vi "Relay Controller.vi"(0 "TSM Context":T2, 7 "Relays":string[](array[string]), 11 "error in":errorcluster) -> (15 "error out":errorcluster)   [LabVIEW 2019]
doc: "This VI is used for toggling 2567, 6368 and 6571 based relays."
uses:
  <vilib>/NI_TestStand_SemiconductorModule/NI_TestStand_Semiconductor_Module.lvlibp/PinMap/General/SemiconductorModuleContext.ctl
  <vilib>/NI_TestStand_SemiconductorModule/NI_TestStand_Semiconductor_Module.lvlibp/1abvi3w/instr.lib/niSwitch/niswitch.llb/niSwitch Relay Action.ctl
  <vilib>/Utility/error.llb/whitespace.ctl
  <vilib>/DAQmx/write.llb/DAQmx Write (Digital 2D Bool NChan 1Samp NLine).vi
  <vilib>/DAQmx/miscellaneous.llb/DAQmx Fill In Error Info.vi
  <vilib>/NI_TestStand_SemiconductorModule/NI_TestStand_Semiconductor_Module.lvlibp
  <instrlib>/niDigital/niDigital.llb/niDigital Write Static Pin State.ctl
  <vilib>/DAQmx/write.llb/DAQmx Write (Digital Bool 1Line 1Point).vi
panel:
  in  "Relay Control":T1=21 caption="relay action (Close Relay)" items=["Open Relay"=20, "Close Relay"=21]
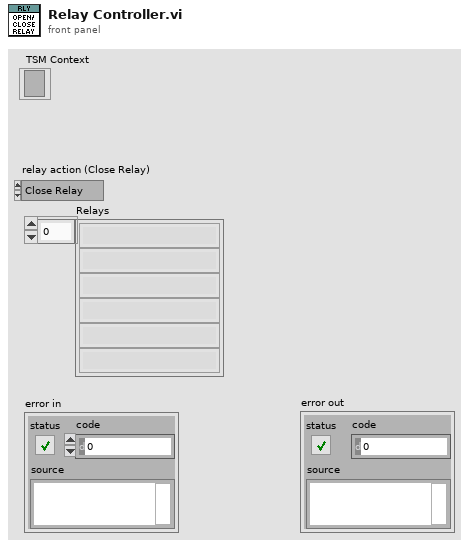
[diagram p1: front panel]
types:
  T1 = typedef "NI_TestStand_Semiconductor_Module.lvlibp/niSwitch Relay Action.ctl" = i32
  T2 = typedef "NI_TestStand_Semiconductor_Module.lvlibp/SemiconductorModuleContext.ctl" = refnum<k7>
  T3 = typedef "whitespace.ctl" = u16
  T4 = typedef "TSM DAQmx Multi-Task.ctl" = cluster{"Pin Query Context":refnum<class "MultiplePinMultipleSessionQueryContext.lvclass">, "SSC":T5[], "Site Numbers":i32[]}
  T5 = typedef "SSC DAQmx.ctl" = cluster{"DAQmx Task ":refnum<k21>, "Channels":string, "Channel Lists":string}
  T6 = typedef "TSM Relay.ctl" = cluster{"TSM Context":T2, "Relays":tag[]}
  T7 = typedef "niDigital Write Static Pin State.ctl" = u8
  T8 = typedef "TSM SSC Digital.ctl" = cluster{"Pin Query Context":refnum<class "DigitalPatternPinQueryContext.lvclass">, "SSC":T9[], "Site Numbers":i32[], "Pins":tag[]}
  T9 = typedef "SSC Digital.ctl" = cluster{"Session":refnum<k15>, "Channel List":string, "Site List":string}
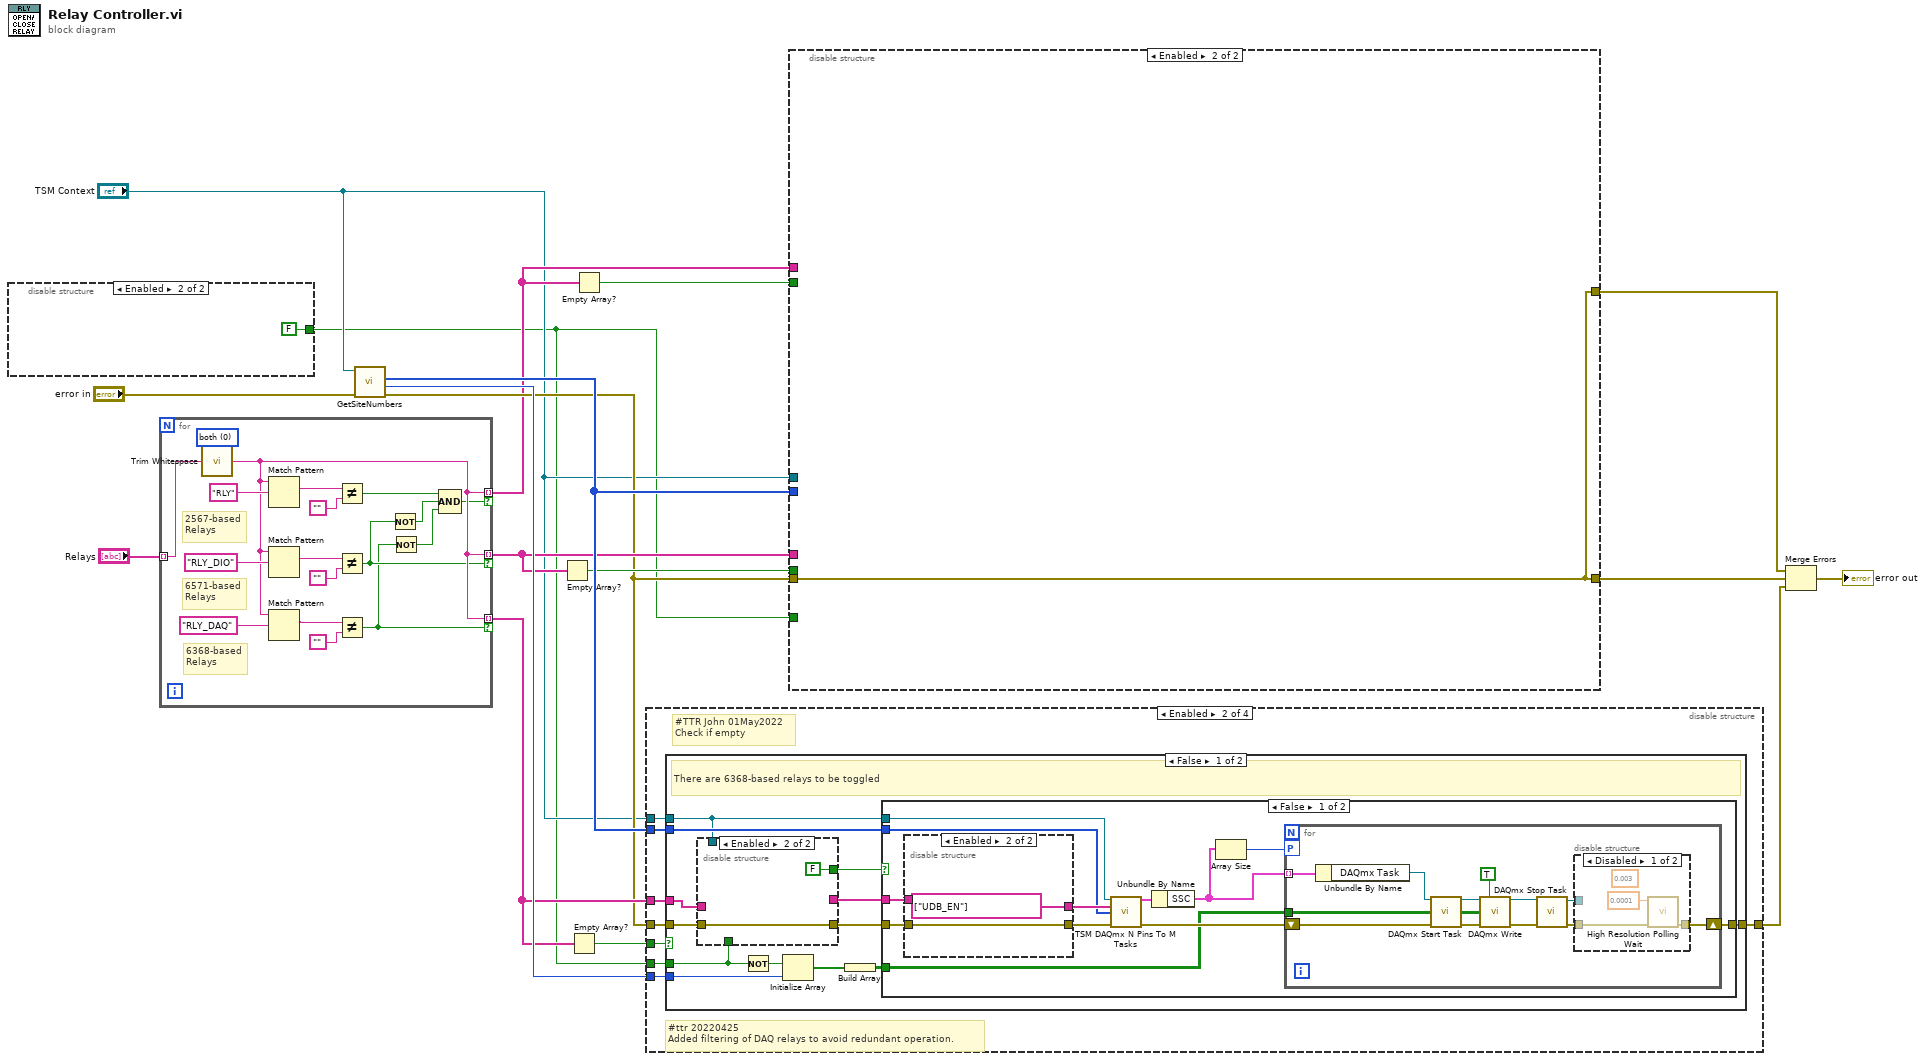
[diagram p0: block diagram]
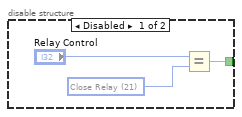
[diagram p2: hidden frame]
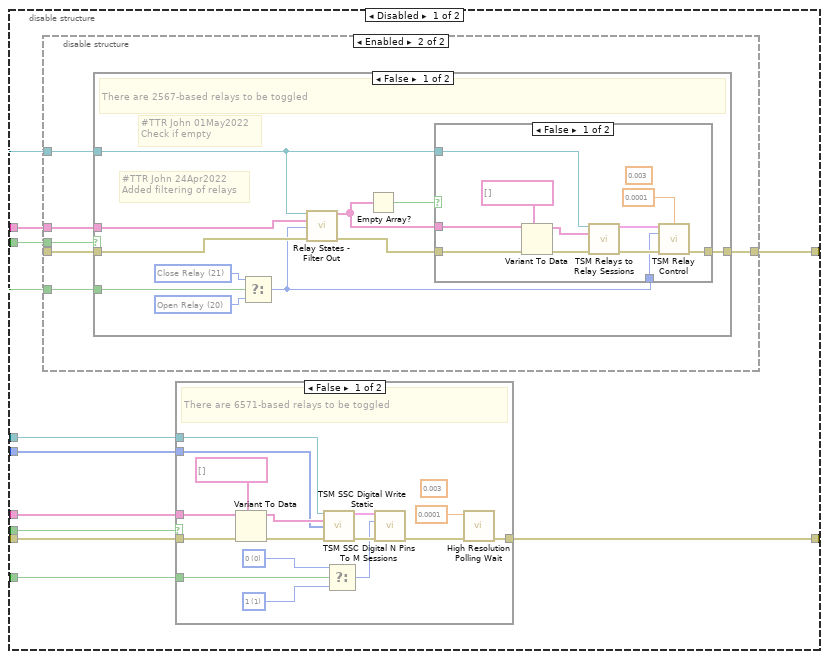
[diagram p3: hidden frame]
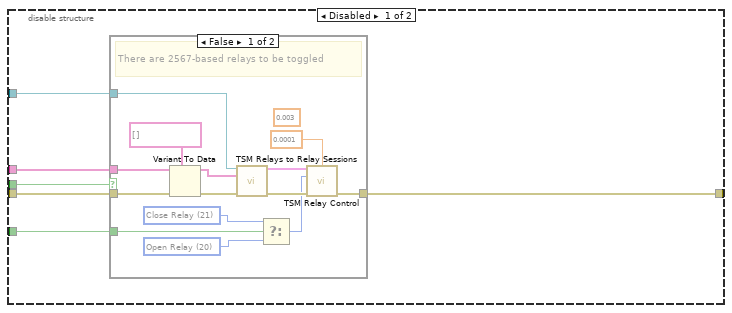
[diagram p4: hidden frame]
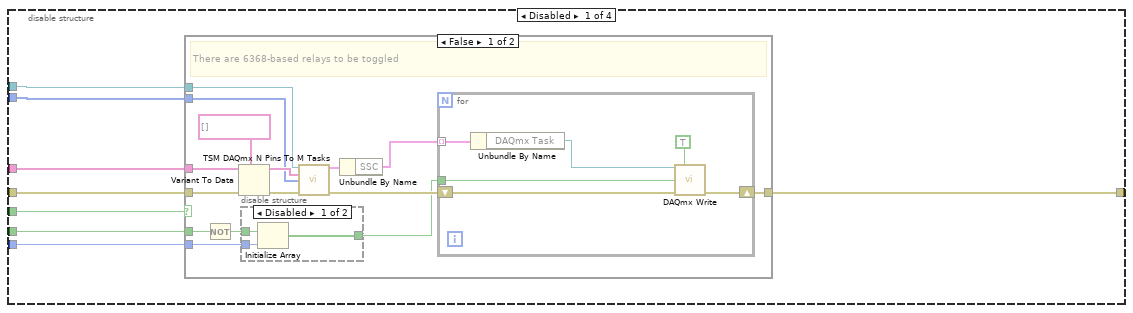
[diagram p9: hidden frame]
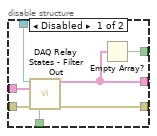
[diagram p12: hidden frame]
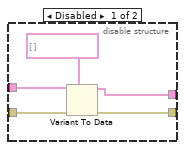
[diagram p13: hidden frame]
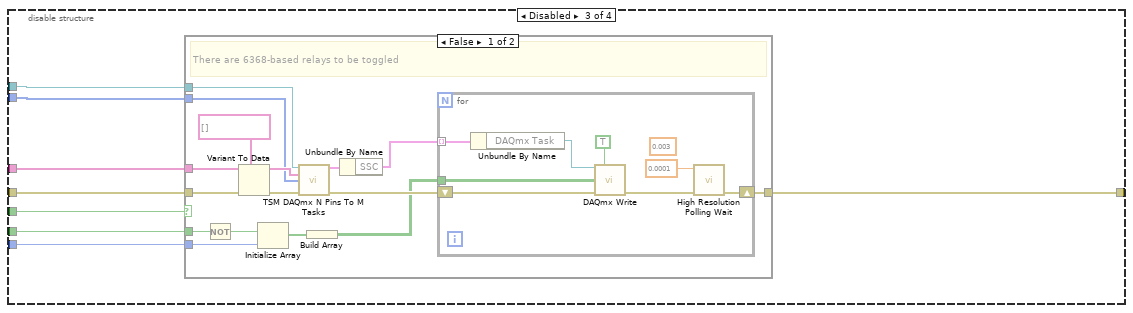
[diagram p17: hidden frame]
diagram:
  n1 = disable-structure shown="Enabled" {
    disable-tunnel: [w20 FALSE] -> w1
    frame Disabled {
      w19 = T1 21 items=["Open Relay"=20, "Close Relay"=21] ("Relay Action")
      n2 = Equal?(x="Relay Control", y=w19) -> (x = y?=w20:bool)
    }
    frame Enabled {
    }
  }
  n3 = for {
    tunnel: "Relays" -> [w30] mode=indexing
    tunnel: [w26] -> w3 mode=indexing if=w24
    tunnel: [w26] -> w9 mode=indexing if=w23
    tunnel: [w26] -> w8 mode=indexing if=w22
    w25 = T3 0 items=["both", "start of string", "end of string"] ("location (both)")
    # "6368-based\nRelays"
    # "6571-based\nRelays"
    # "2567-based\nRelays"
    n4 = call <vilib>:"Trim Whitespace.vi"("string"=w30, "location (both)"=w25) -> ("trimmed string"=w26:string)
    n5 = Match Pattern(string=w26, regular expression="RLY") -> (match substring=w36:string)  [unwired: 1 in, 3 out]
    n6 = Match Pattern(string=w26, regular expression="RLY_DIO") -> (match substring=w33:string)  [unwired: 1 in, 3 out]
    n7 = Match Pattern(string=w26, regular expression="RLY_DAQ") -> (match substring=w31:string)  [unwired: 1 in, 3 out]
    n8 = Not Equal?(x=w36, y="") -> (x != y?=w29:bool)
    n9 = Not Equal?(x=w33, y="") -> (x != y?=w23:bool)
    n10 = Not Equal?(x=w31, y="") -> (x != y?=w22:bool)
    n11 = Not(x=w23) -> (.not. x?=w28:bool)
    n12 = Not(x=w22) -> (.not. x?=w27:bool)
    n13 = Compound Arithmetic op=AND(w29, w28, w27) -> (w24:bool)
  }
  n14 = call <vilib>:"GetSiteNumbers.vi"("error in (no error)"="error in", "Semiconductor Module Context"="TSM Context") -> ("error out"=w5:errorcluster, "Number Of Sites"=w11:i32, "Site Numbers"=w12:i32[])  [unwired: 6 in, 1 out]
  n15 = Empty Array?(array=w9) -> (empty?=w10:bool)
  n16 = Empty Array?(array=w8) -> (empty?=w7:bool)
  n17 = Empty Array?(array=w3) -> (empty?=w4:bool)
  n18 = disable-structure shown="Enabled" {
    disable-tunnel: [w47 w81 w148 _] -> w13
    disable-tunnel: w5 -> [w46 w80 w147 _]
    disable-tunnel: "TSM Context" -> [w45 w79 w146 _]
    disable-tunnel: w12 -> [w44 w78 w145 _]
    disable-tunnel: w11 -> [w43 w77 w144 _]
    disable-tunnel: w8 -> [w42 w76 w143 _]
    disable-tunnel: w7 -> [w41 w75 w142 _]
    disable-tunnel: w1 -> [w40 w74 w141 _]
    frame Disabled {
      n19 = case shown="False" w41 {
        tunnel: w46 -> [w60 w73]
        tunnel: [w61 w73] -> w47
        tunnel: w42 -> [w59 _]
        tunnel: w40 -> [w49 _]
        tunnel: w45 -> [w54 _]
        tunnel: w44 -> [w52 _]
        tunnel: w43 -> [w62 _]
        frame False {
          # "There are 6368-based relays to be toggled"
          n20 = Not(x=w49) -> (.not. x?=w48:bool)
          n21 = Variant To Data(error in=w60, type=tag[] [] ("Pins"), Variant=w59) -> (data=w53:tag[], error out=w57:errorcluster)
          n22 = disable-structure shown="Disabled" {
            disable-tunnel: w62 -> [w65 _]
            disable-tunnel: [w64 w66] -> w51
            disable-tunnel: w48 -> [w63 w66]
            frame Disabled {
              n23 = Initialize Array(w63, w65) -> (w64:bool[])
            }
            frame Enabled {
            }
          }
          n24 = call "TSM DAQmx N Pins To M Tasks.vi"("TSM context"=w54, "Pins"=w53, "Site Numbers"=w52, "error in"=w57) -> ("DAQ TSM Out"=w55:T4, "error out"=w56:errorcluster)  [unwired: 10 in]
          n25 = Unbundle By Name(w55) -> ("SSC"=w50:T5[])
          n26 = for {
            tunnel: w51 -> [w69]
            shift-right: [w72] -> w61
            shift-left: w56 -> [w70]
            tunnel: w50 -> [w68] mode=indexing
            n27 = Unbundle By Name(w68) -> ("DAQmx Task"=w67:refnum<k21>)
            n28 = call-poly <vilib>:"DAQmx Write.vi"("task/channels in"=w67, "auto start"=TRUE, "data"=w69, "error in"=w70) -> ("error out"=w72:errorcluster)  [unwired: 9 in, 2 out]
          }
        }
        frame True {
          # "There are no 6368-based relays to be toggled"
        }
      }
    }
    frame Enabled {
      # "#TTR John 01May2022\nCheck if empty"
      # "#ttr 20220425\nAdded filtering of DAQ relays to avoid redundant operation."
      n29 = case shown="False" w75 {
        tunnel: w80 -> [w92 w140]
        tunnel: [w93 w140] -> w81
        tunnel: w76 -> [w86 _]
        tunnel: w74 -> [w84 _]
        tunnel: w79 -> [w85 _]
        tunnel: w78 -> [w91 _]
        tunnel: w77 -> [w94 _]
        frame False {
          # "There are 6368-based relays to be toggled"
          n30 = disable-structure shown="Enabled" {
            disable-tunnel: w92 -> [w101 w102]
            disable-tunnel: [w100 w102] -> w87
            disable-tunnel: w86 -> [w99 _]
            disable-tunnel: w85 -> [w98 _]
            disable-tunnel: w84 -> [w97 _]
            disable-tunnel: [w96 _] -> w83
            disable-tunnel: [w95 FALSE ("empty?")] -> w82
            frame Disabled {
              n31 = call "DAQ Relay States - Filter Out.vi"("TSM Context"=w98, "RLY in"=w99, "error in (no error)"=w101, "State"=w97) -> ("Relay Filtered out"=w96:string[], "error out"=w100:errorcluster)  [unwired: 10 in]
              n32 = Empty Array?(array=w96) -> (empty?=w95:bool)
            }
            frame Enabled {
            }
          }
          n33 = Not(x=w84) -> (.not. x?=w88:bool)
          n34 = Initialize Array(w88, w94) -> (w90:bool[])
          n35 = Build Array(w90) -> (w89:bool[][])
          n36 = case shown="False" w82 {
            tunnel: [w115 w139] -> w93
            tunnel: w91 -> [w111 _]
            tunnel: w89 -> [w110 _]
            tunnel: w87 -> [w109 w139]
            tunnel: w85 -> [w108 _]
            tunnel: w83 -> [w107 _]
            frame False {
              n37 = disable-structure shown="Enabled" {
                disable-tunnel: [w119 w121] -> w114
                disable-tunnel: [w118 tag[] ["UDB_EN"] ("Pins")] -> w112
                disable-tunnel: w109 -> [w117 w121]
                disable-tunnel: w107 -> [w116 _]
                frame Disabled {
                  n38 = Variant To Data(error in=w117, type=tag[] [] ("Pins"), Variant=w116) -> (data=w118:tag[], error out=w119:errorcluster)
                }
                frame Enabled {
                }
              }
              n39 = call "TSM DAQmx N Pins To M Tasks.vi"("TSM context"=w108, "Pins"=w112, "Site Numbers"=w111, "error in"=w114) -> ("DAQ TSM Out"=w104:T4, "error out"=w113:errorcluster)  [unwired: 10 in]
              n40 = Unbundle By Name(w104) -> ("SSC"=w105:T5[])
              n41 = Array Size(array=w105) -> (size(s)=w106:i32)
              n42 = for {
                tunnel: w110 -> [w134]
                shift-right: [w133] -> w115
                shift-left: w113 -> [w131]
                tunnel: w105 -> [w132] mode=indexing
                workers-P: w106 -> [_]
                n43 = Unbundle By Name(w132) -> ("DAQmx Task"=w123:refnum<k21>)
                n44 = call <vilib>:"DAQmx Start Task.vi"("task/channels in"=w123, "error in"=w131) -> ("task out"=w128:refnum<k21>, "error out"=w129:errorcluster)  [unwired: 12 in]
                n45 = call-poly <vilib>:"DAQmx Write.vi"("task/channels in"=w128, "auto start"=TRUE, "data"=w134, "error in"=w129) -> ("task out"=w127:refnum<k21>, "error out"=w126:errorcluster)  [unwired: 9 in, 1 out]
                n46 = call <vilib>:"DAQmx Stop Task.vi"("task/channels in"=w127, "error in"=w126) -> ("task out"=w124:refnum<k21>, "error out"=w125:errorcluster)  [unwired: 12 in]
                n47 = disable-structure shown="Disabled" {
                  disable-tunnel: [w136 w138] -> w133
                  disable-tunnel: w125 -> [w135 w138]
                  disable-tunnel: w124 -> [_ _]
                  frame Disabled {
                    (unwired) 0.003 ("seconds to wait")
                    n48 = call <vilib>:"High Resolution Polling Wait.vi"("error in (no error)"=w135, "seconds to wait"=0.0001) -> ("error out"=w136:errorcluster)  [unwired: 9 in]
                  }
                  frame Enabled {
                  }
                }
              }
            }
            frame True {
            }
          }
        }
        frame True {
          # "There are no 6368-based relays to be toggled"
        }
      }
    }
    frame Disabled {
      n49 = case shown="False" w142 {
        tunnel: w147 -> [w162 w173]
        tunnel: [w163 w173] -> w148
        tunnel: w143 -> [w161 _]
        tunnel: w141 -> [w150 _]
        tunnel: w146 -> [w156 _]
        tunnel: w145 -> [w154 _]
        tunnel: w144 -> [w164 _]
        frame False {
          # "There are 6368-based relays to be toggled"
          n50 = Not(x=w150) -> (.not. x?=w149:bool)
          n51 = Variant To Data(error in=w162, type=tag[] [] ("Pins"), Variant=w161) -> (data=w155:tag[], error out=w159:errorcluster)
          n52 = Initialize Array(w149, w164) -> (w153:bool[])
          n53 = call "TSM DAQmx N Pins To M Tasks.vi"("TSM context"=w156, "Pins"=w155, "Site Numbers"=w154, "error in"=w159) -> ("DAQ TSM Out"=w157:T4, "error out"=w158:errorcluster)  [unwired: 10 in]
          n54 = Build Array(w153) -> (w152:bool[][])
          n55 = Unbundle By Name(w157) -> ("SSC"=w151:T5[])
          n56 = for {
            tunnel: w152 -> [w170]
            shift-right: [w166] -> w163
            shift-left: w158 -> [w171]
            tunnel: w151 -> [w169] mode=indexing
            (unwired) 0.003 ("seconds to wait")
            n57 = Unbundle By Name(w169) -> ("DAQmx Task"=w168:refnum<k21>)
            n58 = call-poly <vilib>:"DAQmx Write.vi"("task/channels in"=w168, "auto start"=TRUE, "data"=w170, "error in"=w171) -> ("error out"=w165:errorcluster)  [unwired: 9 in, 2 out]
            n59 = call <vilib>:"High Resolution Polling Wait.vi"("error in (no error)"=w165, "seconds to wait"=0.0001) -> ("error out"=w166:errorcluster)  [unwired: 9 in]
          }
        }
        frame True {
          # "There are no 6368-based relays to be toggled"
        }
      }
    }
    frame Disabled {
    }
  }
  n60 = disable-structure shown="Enabled" {
    disable-tunnel: [w183 w252] -> w14
    disable-tunnel: w12 -> [w182 _]
    disable-tunnel: w10 -> [w181 _]
    disable-tunnel: w9 -> [w180 _]
    disable-tunnel: [w179 w252] -> w6
    disable-tunnel: w5 -> [w178 w252]
    disable-tunnel: w4 -> [w177 _]
    disable-tunnel: w3 -> [w176 _]
    disable-tunnel: "TSM Context" -> [w175 _]
    disable-tunnel: w1 -> [w174 _]
    frame Disabled {
      n61 = disable-structure shown="Enabled" {
        disable-tunnel: [w189 w207] -> w179
        disable-tunnel: _ -> [w188 w210]
        disable-tunnel: w175 -> [w187 w208]
        disable-tunnel: w177 -> [w186 w206]
        disable-tunnel: w176 -> [w185 w209]
        disable-tunnel: w174 -> [w184 w205]
        frame Disabled {
          n62 = case shown="False" w186 {
            tunnel: w188 -> [w202 w204]
            tunnel: [w200 w204] -> w189
            tunnel: w187 -> [w203 _]
            tunnel: w185 -> [w201 _]
            tunnel: w184 -> [w194 _]
            frame False {
              (unwired) 0.003 ("Settling Time (s)")
              w192 = T1 20 items=["Open Relay"=20, "Close Relay"=21] ("Relay Action")
              w193 = T1 21 items=["Open Relay"=20, "Close Relay"=21] ("Relay Action")
              # "There are 2567-based relays to be toggled"
              n63 = Variant To Data(error in=w202, type=tag[] [] ("Relays"), Variant=w201) -> (data=w196:tag[], error out=w197:errorcluster)
              n64 = call "TSM Relays to Relay Sessions.vi"("TSM Context"=w203, "Relays"=w196, "error in (no error)"=w197) -> ("TSM Relay Out"=w195:T6, "error out"=w199:errorcluster)  [unwired: 11 in]
              n65 = Select(t=w193, s=w194, f=w192) -> (s? t:f=w191:T1)
              n66 = call "TSM Relay Control.vi"("Relay TSM in"=w195, "Settling Time (s)"=0.0001, "Relay Action"=w191, "error in"=w199) -> ("error out"=w200:errorcluster)  [unwired: 11 in]
            }
            frame True {
              # "There are no 2567-based relays to be toggled"
            }
          }
        }
        frame Enabled {
          n67 = case shown="False" w206 {
            tunnel: w210 -> [w221 w234]
            tunnel: [w220 w234] -> w207
            tunnel: w208 -> [w213 _]
            tunnel: w209 -> [w218 _]
            tunnel: w205 -> [w215 _]
            frame False {
              w217 = T1 20 items=["Open Relay"=20, "Close Relay"=21] ("Relay Action")
              w216 = T1 21 items=["Open Relay"=20, "Close Relay"=21] ("Relay Action")
              # "#TTR John 01May2022\nCheck if empty"
              # "#TTR John 24Apr2022\nAdded filtering of relays"
              # "There are 2567-based relays to be toggled"
              n68 = Select(t=w216, s=w215, f=w217) -> (s? t:f=w214:T1)
              n69 = call "Relay States - Filter Out.vi"("TSM Context"=w213, "RLY in"=w218, "Relay Action in"=w214, "error in (no error)"=w221) -> ("Relay Filtered out"=w212:string[], "error out"=w219:errorcluster)  [unwired: 10 in]
              n70 = Empty Array?(array=w212) -> (empty?=w211:bool)
              n71 = case shown="False" w211 {
                tunnel: [w232 w233] -> w220
                tunnel: w219 -> [w225 w233]
                tunnel: w214 -> [w224 _]
                tunnel: w213 -> [w223 _]
                tunnel: w212 -> [w222 _]
                frame False {
                  (unwired) 0.003 ("Settling Time (s)")
                  n72 = Variant To Data(error in=w225, type=tag[] [] ("Relays"), Variant=w222) -> (data=w228:tag[], error out=w229:errorcluster)
                  n73 = call "TSM Relays to Relay Sessions.vi"("TSM Context"=w223, "Relays"=w228, "error in (no error)"=w229) -> ("TSM Relay Out"=w227:T6, "error out"=w231:errorcluster)  [unwired: 11 in]
                  n74 = call "TSM Relay Control.vi"("Relay TSM in"=w227, "Settling Time (s)"=0.0001, "Relay Action"=w224, "error in"=w231) -> ("error out"=w232:errorcluster)  [unwired: 11 in]
                }
                frame True {
                }
              }
            }
            frame True {
              # "There are no 2567-based relays to be toggled"
            }
          }
        }
      }
      n75 = case shown="False" w181 {
        tunnel: w178 -> [w250 w251]
        tunnel: [w235 w251] -> w183
        tunnel: w180 -> [w249 _]
        tunnel: w175 -> [w246 _]
        tunnel: w182 -> [w243 _]
        tunnel: w174 -> [w239 _]
        frame False {
          (unwired) 0.003 ("seconds to wait")
          w240 = T7 1 items=["0"=0, "1"=1, "X"=5] ("State")
          w241 = T7 0 items=["0"=0, "1"=1, "X"=5] ("State")
          # "There are 6571-based relays to be toggled"
          n76 = Variant To Data(error in=w250, type=tag[] [] ("data"), Variant=w249) -> (data=w245:tag[], error out=w248:errorcluster)
          n77 = call "TSM SSC Digital N Pins To M Sessions.vi"("TSM context"=w246, "Pins"=w245, "Site Numbers"=w243, "error in"=w248) -> ("Digital TSM Out"=w242:T8, "error out"=w247:errorcluster)  [unwired: 10 in]
          n78 = Select(t=w241, s=w239, f=w240) -> (s? t:f=w238:T7)
          n79 = call "TSM SSC Digital Write Static.vi"("Digital TSM in"=w242, "State"=w238, "error in"=w247) -> ("error out"=w236:errorcluster)  [unwired: 11 in, 1 out]
          n80 = call <vilib>:"High Resolution Polling Wait.vi"("error in (no error)"=w236, "seconds to wait"=0.0001) -> ("error out"=w235:errorcluster)  [unwired: 9 in]
        }
        frame True {
          # "There are no 2567-based relays to be toggled"
        }
      }
    }
    frame Enabled {
    }
  }
  n81 = Merge Errors(w6, w14, w13) -> (→"error out":errorcluster)
